vi "ConvertConditions.vi"(3 "metric ids":string[](array[string]), 4 "conditions":T1[](array[typedef])) -> (0 "valid config":bool, 1 "trigger conditions":T2[](array[typedef]))   [LabVIEW 2017, in "OpState.lvlib"]
uses:
  <vilib>/addons/InsightCM/Devices/Shared/Common/OpState/OpState.lvlib
  <vilib>/addons/InsightCM/Devices/Shared/Common/Trigger/controls/TriggerCondition.ctl
  <vilib>/addons/InsightCM/MessageBus/Base/controls/Condition.ctl
  <vilib>/addons/InsightCM/Devices/Shared/Common/Trigger/Trigger.lvlib
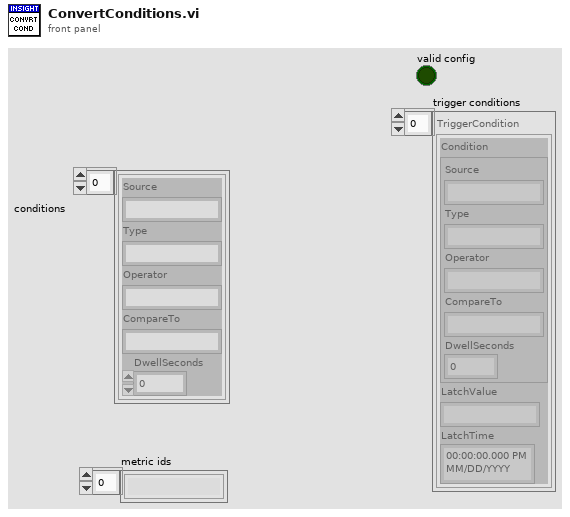
[diagram p1: front panel]
types:
  T1 = typedef "Condition.ctl" = cluster{"Source":string, "Type":string, "Operator":string, "CompareTo":string, "DwellSeconds":dbl}
  T2 = typedef "Trigger.lvlib/TriggerCondition.ctl" = cluster{"Condition":T1, "LatchValue":string, "LatchTime":timestamp}
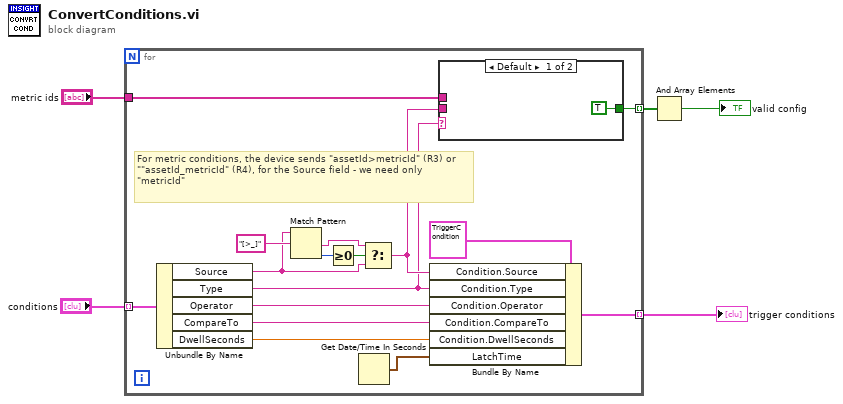
[diagram p0: block diagram]
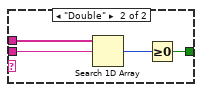
[diagram p2: hidden frame]
diagram:
  n1 = for {
    tunnel: "conditions" -> [w12] mode=indexing
    tunnel: [w11] -> w5 mode=indexing
    tunnel: "metric ids" -> [w9]
    tunnel: [w7] -> w2 mode=indexing
    # "For metric conditions, the device sends \"assetId>metricId\" (R3) or \"\"assetId_metricId\" (R4), for the Source field - we need only \"metricId\""
    n2 = Unbundle By Name(w12) -> ("Source"=w13:string, "Type"=w6:string, "Operator"=w20:string, "CompareTo"=w19:string, "DwellSeconds"=w18:dbl)
    n3 = Match Pattern(string=w13, regular expression="[>_]") -> (after substring=w14:string, offset past match=w16:i32)  [unwired: 1 in, 2 out]
    n4 = Greater Or Equal To 0?(x=w16) -> (x >= 0?=w15:bool)
    n5 = Get Date/Time In Seconds() -> (seconds since 1Jan1904=w10:timestamp)
    n6 = Select(t=w14, s=w15, f=w13) -> (s? t:f=w8:string)
    n7 = Bundle By Name(cluster=T2 {"Condition"={"Source"="", "Type"="", "Operator"="", "CompareTo"="", "DwellSeconds"=0.0}, "LatchValue"="", "LatchTime"=timestamp(0 s since 1904-01-01)} ("TriggerCondition"), "Condition.Source"=w8, "Condition.Type"=w6, "Condition.Operator"=w20, "Condition.CompareTo"=w19, "Condition.DwellSeconds"=w18, "LatchTime"=w10) -> (w11:T2)
    n8 = case shown="Default" w6 {
      tunnel: w9 -> [_ w26]
      tunnel: w8 -> [_ w25]
      tunnel: [TRUE w23] -> w7
      frame Default {
      }
      frame "Double" {
        n9 = Search 1D Array(1D array=w26, element=w25) -> (index of element=w24:i32)  [unwired: 1 in]
        n10 = Greater Or Equal To 0?(x=w24) -> (x >= 0?=w23:bool)
      }
    }
  }
  "trigger conditions" <- w5
  n11 = And Array Elements(Boolean array=w2) -> (logical AND=→"valid config":bool)
